vi "EnqueueEvents.vi"(1 "data":variant, 2 "message":string) -> ()   [LabVIEW 2011]
uses:
  event.ctl
  Global.vi
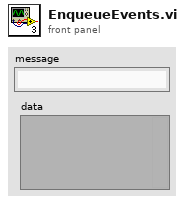
[diagram p1: front panel]
types:
  T1 = typedef "event.ctl" = cluster{"message":string, "data":variant}
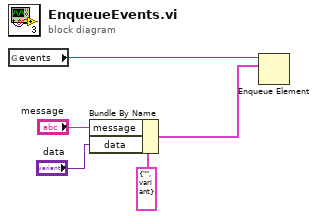
[diagram p0: block diagram]
diagram:
  n1 = global read "Global.vi" "events"() -> (w3:refnum<queue>)
  n2 = Bundle By Name(cluster=T1 {"message"="", "data"=variant} ("element"), "message"="message", "data"="data") -> (w1:T1)
  n3 = Enqueue Element(queue=w3, element=w1) -> ()  [unwired: 2 in, 3 out]
